vi "niRFUtil FTW FFT (real wfm).vi"(3 "Padding (1)":T1=1.0 min=1.0 format="%.2f", 5 "Waveform In (V)":T4 {"y" min=0 max=127 format="%.2f"; "dx" format="%^.2e"; "x0" format="%^.2e"}) -> (0 "-ENBW (dB-Hz)":sgl format="%.2f", 1 "Coherent Loss (dB)":sgl format="%.2f", 2 "Waveform Out (V)":T2 {"y" format="%.2f"; "dx" format="%^.2e"; "x0" format="%^.2e"})   [LabVIEW 2015, in "niRFUtil.lvlib"]
doc: "(c) Copyright 2006, National Instruments, Inc. This VI may not be duplicated, sold, or distributed without written consent from National Instruments."
uses:
  niRFUtil.lvlib
  Includes/niRFUtil INC Real Waveform.ctl
  Includes/niRFUtil INC Real Array.ctl
  Includes/niRFUtil INC Complex Waveform.ctl
  Includes/niRFUtil INC Complex Array.ctl
  Includes/niRFUtil INC FFT Padding.ctl
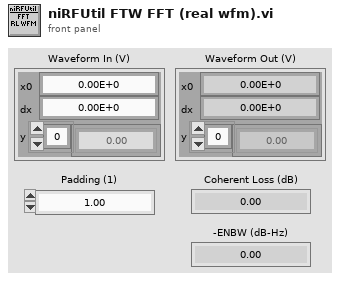
[diagram p1: front panel]
types:
  T1 = typedef "niRFUtil.lvlib/niRFUtil INC FFT Padding.ctl" = dbl
  T2 = typedef "niRFUtil.lvlib/niRFUtil INC Complex Waveform.ctl" = cluster{"x0":dbl, "dx":dbl, "y":T3}
  T3 = typedef "niRFUtil.lvlib/niRFUtil INC Complex Array.ctl" = csg[]
  T4 = typedef "niRFUtil.lvlib/niRFUtil INC Real Waveform.ctl" = cluster{"x0":dbl, "dx":dbl, "y":T5}
  T5 = typedef "niRFUtil.lvlib/niRFUtil INC Real Array.ctl" = sgl[]
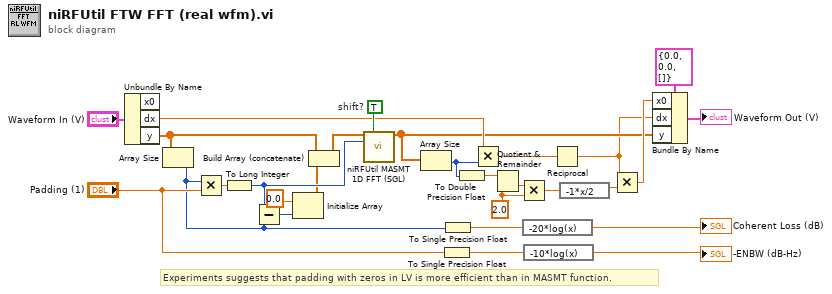
[diagram p0: block diagram]
diagram:
  w19 = 2.0 ("y")
  w24 = TRUE  # shift?
  # "Experiments suggests that padding with zeros in LV is more efficient than in MASMT function."
  n1 = Unbundle By Name("Waveform In (V)") -> ("dx"=w18:dbl, "y"=w3:T5)  [unwired: 1 out]
  n2 = Array Size(array=w3) -> (size(s)=w7:i32)
  n3 = Multiply(x=w7, y="Padding (1)") -> (x*y=w13:T1)
  n4 = To Long Integer(number=w13) -> (32bit integer=w8:i32)
  n5 = Subtract(x=w8, y=w7) -> (x-y=w6:i32)
  n6 = Initialize Array(sgl 0.0, w6) -> (w4:sgl[])
  n7 = Build Array (concatenate)(w3, w4) -> (w2:T5)
  n8 = call "niRFUtil MASMT 1D FFT (SGL).vi"("X"=w2, "shift?"=w24, "FFT size"=w8) -> ("FFT {X}"=w16:csg[])  [unwired: 11 in, 1 out]
  n9 = Array Size(array=w16) -> (size(s)=w15:i32)
  n10 = To Single Precision Float(number="Padding (1)") -> (single precision float=w1:sgl)
  n11 = To Single Precision Float(number=w7) -> (single precision float=w12:sgl)
  n12 = To Double Precision Float(number=w15) -> (double precision float=w14:dbl)
  n13 = Multiply(x=w18, y=w15) -> (x*y=w23:dbl)
  n14 = Quotient & Remainder(x=w14, y=w19) -> (floor(x/y)=w21:dbl)  [unwired: 1 out]
  n15 = Multiply(x=w21, y=w19) -> (x*y=w20:dbl)
  n16 = expression code="-20*log(x)"(w12) -> (→"Coherent Loss (dB)":sgl)
  n17 = expression code="-10*log(x)"(w1) -> (→"-ENBW (dB-Hz)":sgl)
  n18 = Reciprocal(x=w23) -> (1/x=w11:dbl)
  n19 = expression code="-1*x/2"(w20) -> (w22:dbl)
  n20 = Multiply(x=w11, y=w22) -> (x*y=w17:dbl)
  n21 = Bundle By Name(cluster=T2 {"x0"=0.0, "dx"=0.0, "y"=[]} ("Complex Waveform"), "x0"=w17, "dx"=w11, "y"=w16) -> (→"Waveform Out (V)":T2)
